vi "addChild.vi"(0 "reference":refnum<class "AbstractNode.lvclass">, 1 "node":refnum<class "AbstractNode.lvclass">, 2 "index(last)":i32=-1, 5 "error in (no error)":errorcluster) -> (14 "reference out":refnum<class "AbstractNode.lvclass">, 19 "error out":errorcluster)   [LabVIEW 2014, in "AbstractNode.lvclass"]
doc: "public void addChild(int index, Node node)"
uses:
  <resource>/Framework/Providers/Open_GDS/UML/AbstractNode_class/AbstractNode.lvclass
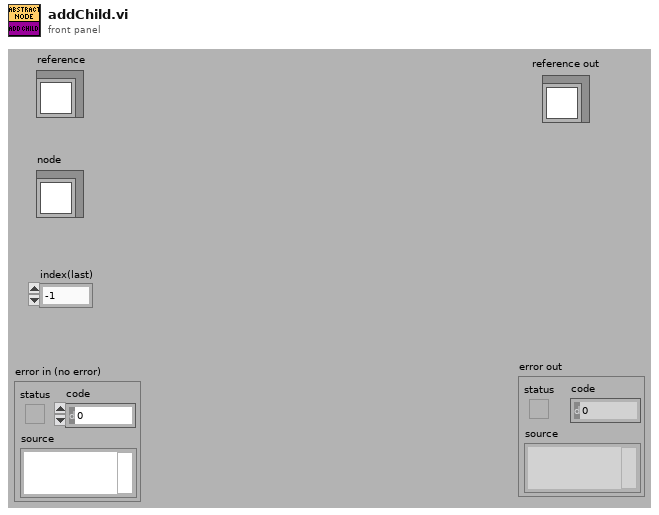
[diagram p1: front panel]
types:
  T1 = typedef "AbstractNode.lvclass/ObjectAttributes.ctl" = cluster{"parent":refnum<class "AbstractNode.lvclass">, "children":refnum<class "AbstractNode.lvclass">[], "Hidden":bool}
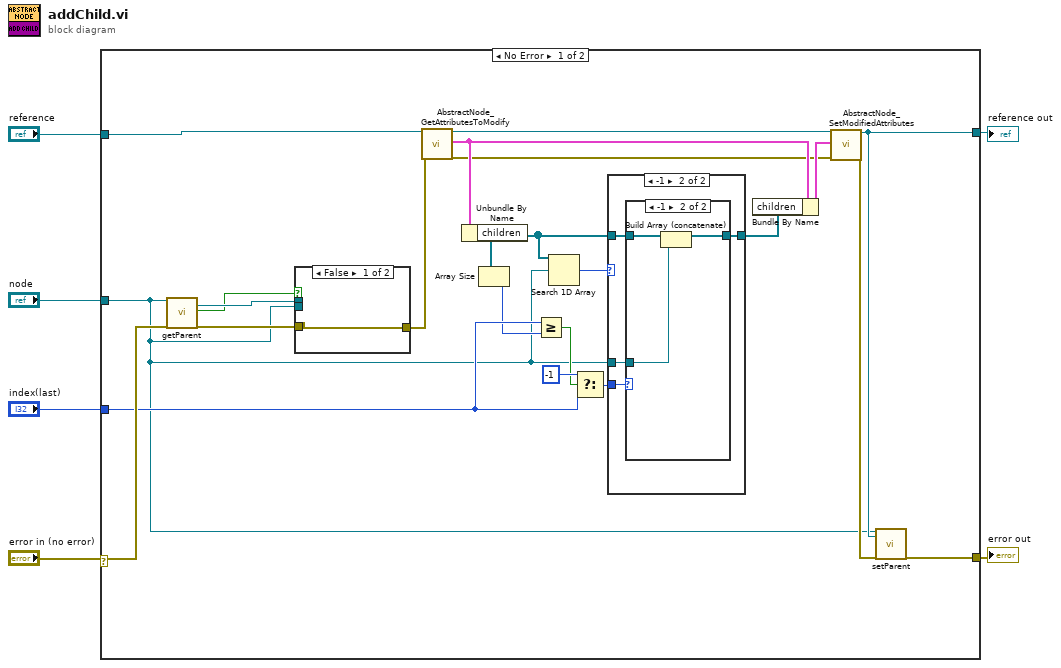
[diagram p0: block diagram]
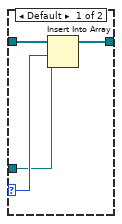
[diagram p3: hidden frame]
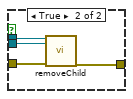
[diagram p4: hidden frame]
diagram:
  n1 = case shown="No Error" "error in (no error)" {
    selector: "error in (no error)" -> [w25 w46]
    tunnel: "reference" -> [w28 w47]
    tunnel: [w27 w46] -> w5
    tunnel: [w26 w47] -> w4
    tunnel: "node" -> [w8 _]
    tunnel: "index(last)" -> [w24 _]
    frame No Error {
      n2 = call-dynamic "getParent.vi"("reference"=w8, "error in (no error)"=w25) -> ("parentNode"=w11:refnum<class "AbstractNode.lvclass">, "ValidParent"=w10:bool, "error out"=w21:errorcluster)  [unwired: 13 in, 2 out]
      n3 = case shown="False" w10 {
        tunnel: w21 -> [w41 w45]
        tunnel: w11 -> [_ w44]
        tunnel: w8 -> [_ w43]
        tunnel: [w41 w42] -> w20
        frame False {
        }
        frame True {
          n4 = call-dynamic "removeChild.vi"("reference"=w44, "node"=w43, "error in (no error)"=w45) -> ("error out"=w42:errorcluster)  [unwired: 15 in, 1 out]
        }
      }
      n5 = call <resource>:"AbstractNode_GetAttributesToModify.vi"("reference in"=w28, "error in (no error)"=w20) -> ("reference out"=w18:refnum<class "AbstractNode.lvclass">, "Attributes"=w19:T1, "error out"=w17:errorcluster)  [unwired: 1 in, 14 out]
      n6 = Unbundle By Name(w19) -> ("children"=w9:refnum<class "AbstractNode.lvclass">[])
      n7 = Array Size(array=w9) -> (size(s)=w13:i32)
      n8 = Greater Or Equal?(x=w24, y=w13) -> (x >= y?=w12:bool)
      n9 = Search 1D Array(1D array=w9, element=w8) -> (index of element=w7:i32)  [unwired: 1 in]
      n10 = Select(t=-1, s=w12, f=w24) -> (s? t:f=w15:i32)
      n11 = case shown="-1" w7 {
        tunnel: [w29 w33] -> w22
        tunnel: w15 -> [_ w32]
        tunnel: w9 -> [w29 w31]
        tunnel: w8 -> [_ w30]
        frame Default {
        }
        frame -1 {
          n12 = case shown="-1" w32 {
            selector: w32 -> [w35 _]
            tunnel: w31 -> [w37 w40]
            tunnel: [w36 w38] -> w33
            tunnel: w30 -> [w34 w39]
            frame Default {
              n13 = Insert Into Array(array=w37, index=w35, new element=w34) -> (w36:refnum<class "AbstractNode.lvclass">[])
            }
            frame -1 {
              n14 = Build Array (concatenate)(w40, w39) -> (w38:refnum<class "AbstractNode.lvclass">[])
            }
          }
        }
      }
      n15 = Bundle By Name(cluster=w19, "children"=w22) -> (w23:T1)
      n16 = call <resource>:"AbstractNode_SetModifiedAttributes.vi"("reference in"=w18, "Attributes"=w23, "error in (no error)"=w17) -> ("reference out"=w26:refnum<class "AbstractNode.lvclass">, "error out"=w16:errorcluster)  [unwired: 3 in, 12 out]
      n17 = call-dynamic "setParent.vi"("reference"=w8, "node"=w26, "error in (no error)"=w16) -> ("error out"=w27:errorcluster)  [unwired: 15 in, 1 out]
    }
    frame Error {
    }
  }
  "reference out" <- w4
  "error out" <- w5
